vi "LJM_ByteArrayToUINT16.vi"(1 "Byte Array":u8[](array[numeric])) -> (0 "U16":u16)   [LabVIEW 2020]
panel:
  # "Converts the first 2 elements of a big-endian byte array to a U16"
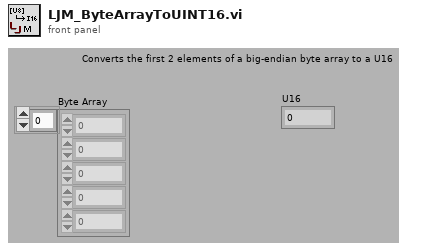
[diagram p1: front panel]
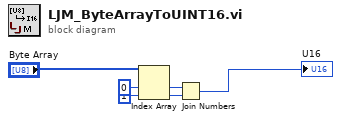
[diagram p0: block diagram]
diagram:
  n1 = Index Array(array="Byte Array", index #1=0 ("Index"), index #2=1 ("Index")) -> (element #1=w2:u8, element #2=w3:u8)
  n2 = Join Numbers(hi=w2, lo=w3) -> ((hi.lo)=→"U16":u16)
